vi "Send Packet.vi"(8 "error in (no error)":errorcluster, 10 "Packet":string, 11 "StatD Interface in":refnum<class "StatD Interface.lvclass">) -> (0 "error out":errorcluster, 3 "StatD Interface out":refnum<class "StatD Interface.lvclass">)   [LabVIEW 2011, in "StatD Interface.lvclass"]
doc: "Sends the UDP packet to the aggregator."
uses:
  StatD Interface.lvclass
  StatD Interface.lvclass/StatD Interface.ctl
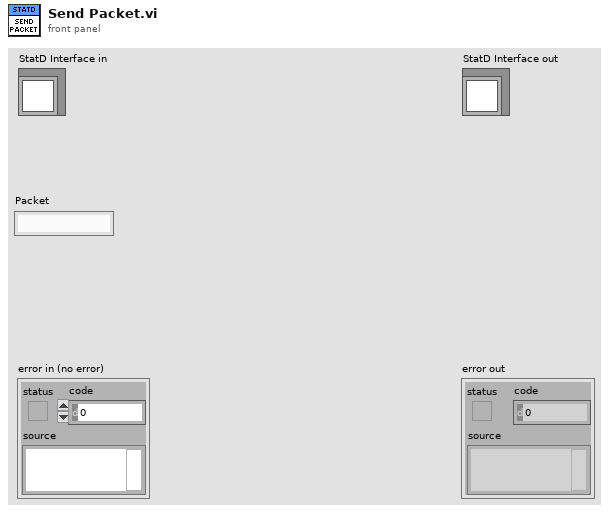
[diagram p1: front panel]
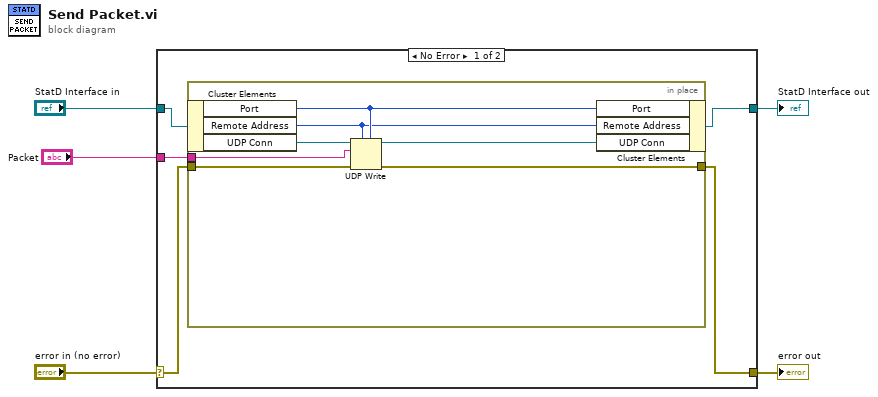
[diagram p0: block diagram]
diagram:
  n1 = case shown="No Error" "error in (no error)" {
    selector: "error in (no error)" -> [w8 w19]
    tunnel: [w6 w19] -> w4
    tunnel: [w9 w18] -> w2
    tunnel: "StatD Interface in" -> [w10 w18]
    tunnel: "Packet" -> [w7 _]
    frame No Error {
      n2 = in-place {
        in-place-border: w8 -> [w13]
        in-place-border: w7 -> [w12]
        in-place-border: [w11] -> w6
        n3 = in-place-cluster #1(w10) -> ("Port"=w15:u16, "Remote Address"=w14:u32, "UDP Conn"=w17:refnum<k16>)
        n4 = UDP Write(address=w14, port or service name=w15, connection ID=w17, data in=w12, 8:w13) -> (error out=w11:errorcluster, 3:w16:refnum<k16>)  [unwired: 1 in]
        n5 = in-place-cluster #1("Port"=w15, "Remote Address"=w14, "UDP Conn"=w16) -> (w9:refnum<class "StatD Interface.lvclass">)
      }
    }
    frame Error {
    }
  }
  "error out" <- w4
  "StatD Interface out" <- w2
